vi "Select System SAL.vi"(8 "error in (no error)":errorcluster, 11 "System Health Module in":refnum<class "System Health Module.lvclass">) -> (0 "error out":errorcluster, 3 "System Health Module out":refnum<class "System Health Module.lvclass">)   [LabVIEW 2020, in "Volatus.lvlib" / "System Health Module.lvclass"]
uses:
  System Health Module.lvclass
  System Health Module.lvclass/System Health Module.ctl
  Windows System SAL/Windows System SAL.lvclass
  Linux System SAL/Linux System SAL.lvclass
  System SAL/System SAL.lvclass
  C:/dev/lv20CE/relink/lv-volatus/Volatus/Windows System SAL/Windows System SAL.lvclass
  C:/dev/lv20CE/relink/lv-volatus/Volatus/System SAL/System SAL.lvclass
  C:/dev/lv20CE/relink/lv-volatus/Volatus/Linux System SAL/Linux System SAL.lvclass
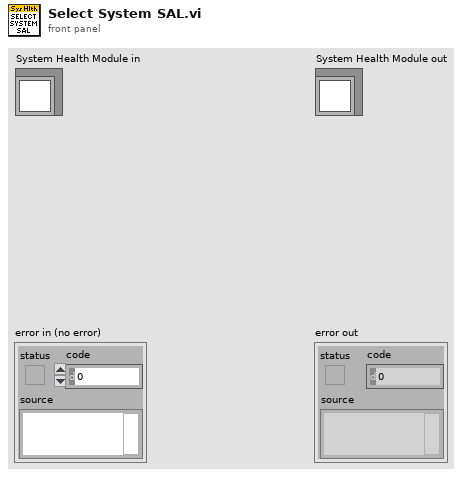
[diagram p1: front panel]
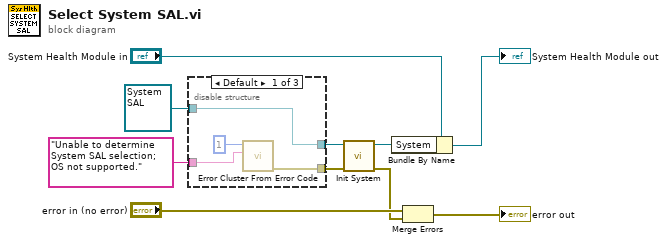
[diagram p0: block diagram]
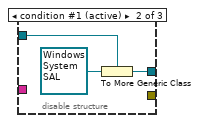
[diagram p2: hidden frame]
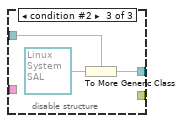
[diagram p3: hidden frame]
diagram:
  n1 = disable-structure shown="Default" {
    disable-tunnel: [w12 w16 w19] -> w2
    disable-tunnel: "Unable to determine System SAL selection; OS not supported." -> [w13 _ _]
    disable-tunnel: refnum<class "System SAL.lvclass"> refnum ("Volatus:System SAL.lvclass") -> [w12 w15 w18]
    disable-tunnel: [w11 _ _] -> w4
    frame condition #0 {
      n2 = call <vilib>:"Error Cluster From Error Code.vi"("error message (\"\")"=w13, "error code (0)"=1) -> ("error out"=w11:errorcluster)  [unwired: 7 in]
    }
    frame condition #1 (active) {
      n3 = To More Generic Class(target class=w15, reference=refnum<class "Windows System SAL.lvclass"> refnum ("Volatus:Windows System SAL.lvclass")) -> (generic class reference=w16:refnum<class "System SAL.lvclass">)
    }
    frame condition #2 {
      n4 = To More Generic Class(target class=w18, reference=refnum<class "Linux System SAL.lvclass"> refnum ("Volatus:Linux System SAL.lvclass")) -> (generic class reference=w19:refnum<class "System SAL.lvclass">)
    }
  }
  n5 = call-dynamic "Init System.vi"("error in (no error)"=w4, "System SAL in"=w2) -> ("error out"=w3:errorcluster, "System SAL out"=w1:refnum<class "System SAL.lvclass">)  [unwired: 8 in]
  n6 = Bundle By Name(cluster="System Health Module in", "System"=w1) -> (→"System Health Module out":refnum<class "System Health Module.lvclass">)
  n7 = Merge Errors("error in (no error)", w3) -> (→"error out":errorcluster)
